vi "IP Dialog.vi"(8 "error in (no error)":errorcluster, 11 "UDP_Service in":refnum<class "UDP_Service.lvclass">) -> (0 "error out":errorcluster, 3 "UDP_Service out":refnum<class "UDP_Service.lvclass">)   [LabVIEW 2016, in "CoreAssertAPI.lvlib" / "UDP_Service.lvclass"]
doc: "Dialog box to allow the user to input an IP address.\nIf the dialog is cancelled - error 43 is output which prevents the actor module from loading."
uses:
  UDP_Service.lvclass
  UDP_Service.lvclass/UDP_Service.ctl
panel:
  in  "LOCALHOST":bool
  in  "OK":bool
  in  "IP Address":string
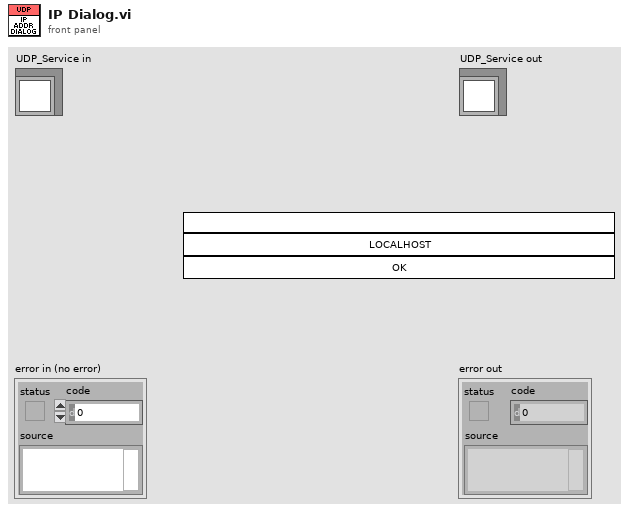
[diagram p1: front panel]
types:
  T1 = enum32{"Invalid", "Standard", "Closed", "Hidden", "Minimized", "Maximized"}
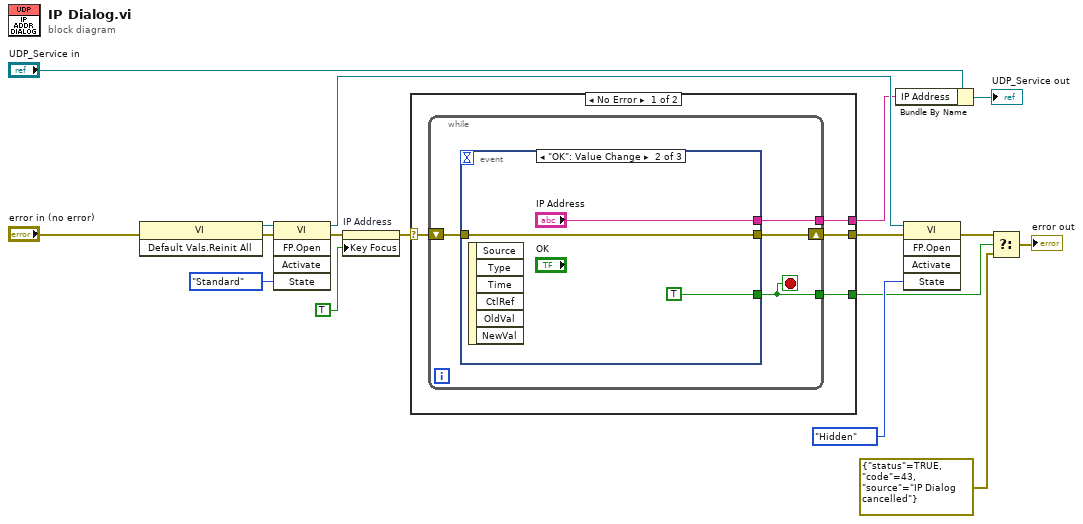
[diagram p0: block diagram]
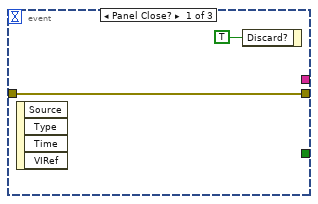
[diagram p2: hidden frame]
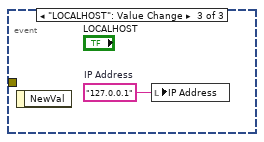
[diagram p3: hidden frame]
diagram:
  n1 = invoke class="VI" method="Default Vals.Reinit All"(error in="error in (no error)") -> (reference out=w14:refnum<vi>, error out=w15:errorcluster)  [unwired: 2 in, 1 out]
  n2 = invoke class="VI" method="FP.Open"(reference=w14, error in=w15, "State"=T1."Standard") -> (reference out=w10:refnum<vi>, error out=w12:errorcluster)  [unwired: 2 in, 3 out]
  n3 = property on="IP Address" class="Str"(error in=w12, "Key Focus"=TRUE) -> (error out=w2:errorcluster)  [unwired: 1 in, 1 out]
  n4 = case shown="No Error" w2 {
    selector: w2 -> [w19 w32]
    tunnel: [w21 _] -> w3
    tunnel: [w20 _] -> w8
    tunnel: [w18 w32] -> w11
    frame No Error {
      n5 = while {
        tunnel: [w25] -> w21
        tunnel: [w22] -> w20
        shift-right: [w23] -> w18
        shift-left: w19 -> [w24]
        stop <- w22 stop-if-true
        n6 = event shown="[1] \"OK\": Value Change" {
          selector: _ -> [_ _ _]
          dyn-events: _ -> [_ _ _]
          timeout: _ -> [_ _ _]
          tunnel: [_ "IP Address" _] -> w25
          tunnel: [_ TRUE _] -> w22
          tunnel: w24 -> [w26 w28 _]
          tunnel: [w26 w28 _] -> w23
          event Panel Close? {
            n7 = event-data() -> ()  [unwired: 1 in, 4 out]
            n8 = event-data("Discard?"=TRUE) -> ()  [unwired: 1 in, 1 out]
          }
          event "OK": Value Change {
            n9 = event-data() -> ()  [unwired: 1 in, 6 out]
          }
          event "LOCALHOST": Value Change {
            w31 = "127.0.0.1"  # IP Address
            n10 = event-data() -> ()  [unwired: 1 in, 1 out]
            n11 = local write "IP Address"(w31) -> ()
          }
        }
      }
    }
    frame Error {
    }
  }
  n12 = Bundle By Name(cluster="UDP_Service in", "IP Address"=w3) -> (→"UDP_Service out":refnum<class "UDP_Service.lvclass">)
  n13 = invoke class="VI" method="FP.Open"(reference=w10, error in=w11, "State"=T1."Hidden") -> (error out=w7:errorcluster)  [unwired: 2 in, 4 out]
  n14 = Select(t=w7, s=w8, f=errorcluster {"status"=TRUE, "code"=43, "source"="IP Dialog cancelled"}) -> (s? t:f=→"error out":errorcluster)
